vi "ROI grp-Add new POIs to the table.vi"(8 "error in (no error)":errorcluster, 11 "New POI indexes":i32[](array[numeric])) -> (0 "error out":errorcluster, 3 "reference out":refnum<vi>)   [LabVIEW 2020]
uses:
  Globals/gl_ROI grp window globals.vi
  <userlib>/_OpenG.lib/array/array.llb/Search 1D Array (String)__ogtk.vi
  <userlib>/_OpenG.lib/array/array.llb/Delete Elements from 1D Array (String)__ogtk.vi
panel:
  out "New number of rows":i32
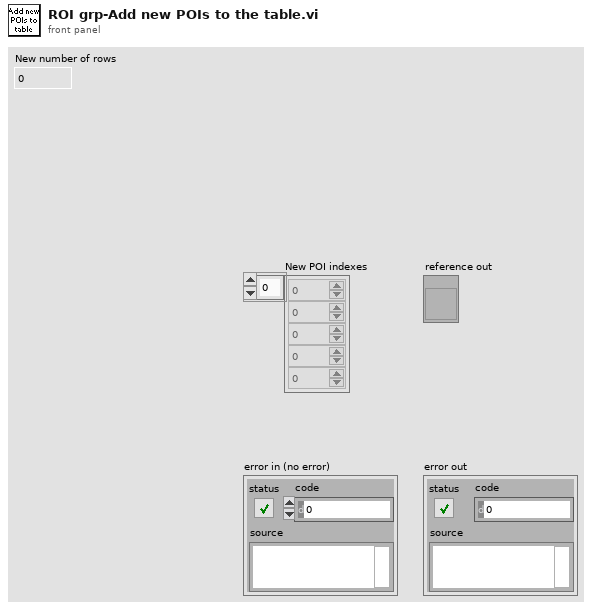
[diagram p1: front panel]
types:
  T1 = typedef "ROI grp-window ctrl refs.ctl" = cluster{"This VI":refnum<vi>, "Pane":refnum<vi>, "Table":refnum<vi>}
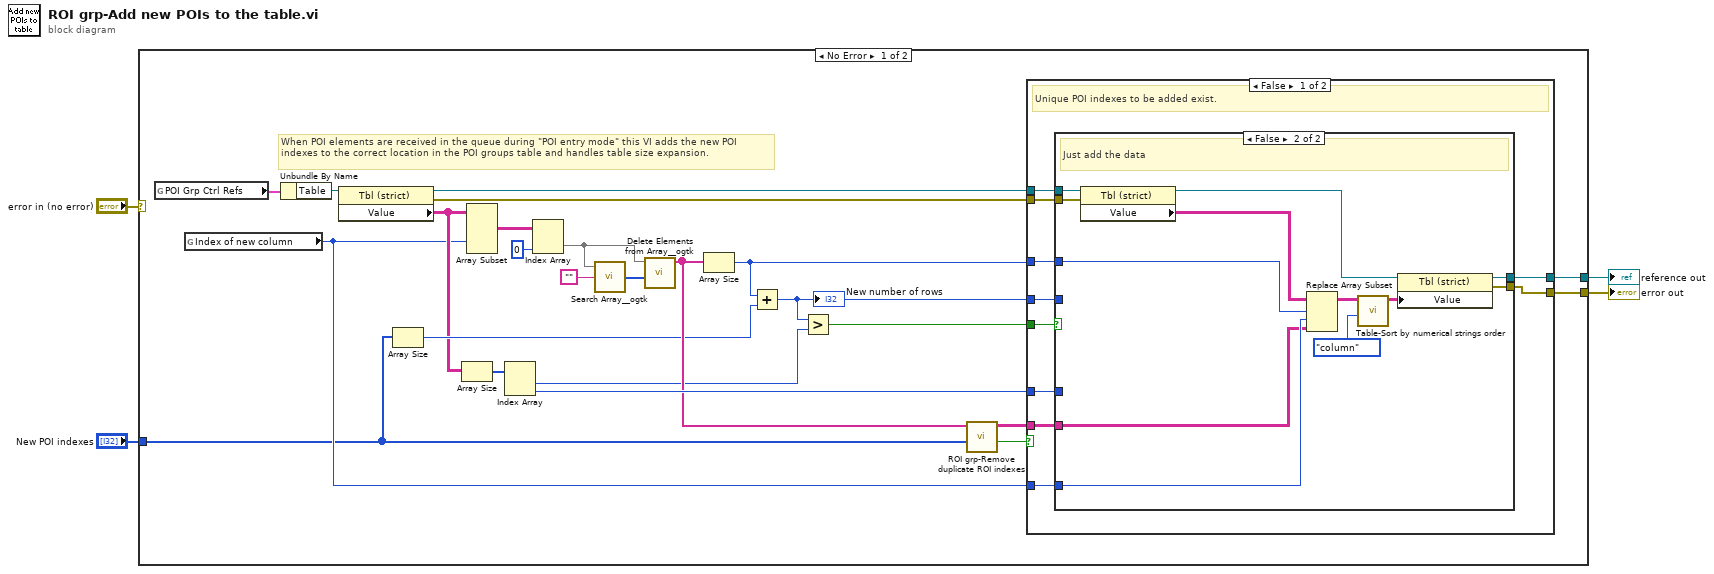
[diagram p0: block diagram]
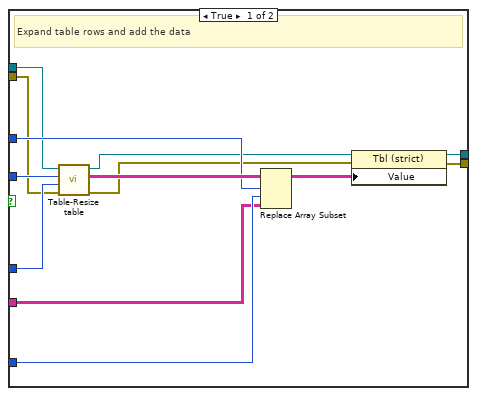
[diagram p2: hidden frame]
diagram:
  n1 = case shown="No Error" "error in (no error)" {
    selector: "error in (no error)" -> [_ w66]
    tunnel: [w11 _] -> w4
    tunnel: [w9 w66] -> w3
    tunnel: "New POI indexes" -> [w7 _]
    frame No Error {
      # "When POI elements are received in the queue during \"POI entry mode\" this VI adds the new POI indexes to the correct location in the POI groups table and handles table size expansion."
      n2 = global read "gl_ROI grp window globals.vi" "POI Grp Ctrl Refs"() -> (w5:T1)
      n3 = global read "gl_ROI grp window globals.vi" "Index of new column"() -> (w10:i32)
      n4 = Unbundle By Name(w5) -> ("Table"=w13:refnum<vi>)
      n5 = property class="Tbl (strict)"(reference=w13) -> (reference out=w12:refnum<vi>, error out=w14:errorcluster, "Value"=w17:string[][])  [unwired: 1 in]
      n6 = Array Size(array=w7) -> (size(s)=w21:i32)
      n7 = Array Size(array=w17) -> (size(s)=w26:i32[])
      n8 = Array Subset(array=w17, index (col)=w10) -> (w25:string[][])  [unwired: 3 in]
      n9 = Index Array(array=w26) -> (element #1=w20:i32, element #2=w28:i32)  [unwired: 2 in]
      n10 = Index Array(array=w25, index (col)=0 ("disabled index (col)")) -> (element=w16:string[])  [unwired: 1 in]
      n11 = call-poly <userlib>:"Search Array__ogtk.vi"("Array"=w16, "Element Data"="") -> ("Indices of Elements"=w23:i32[])  [unwired: 7 in]
      n12 = call-poly <userlib>:"Delete Elements from Array__ogtk.vi"("indices"=w23, "array"=w16) -> ("array w/ subset deleted"=w27:string[])  [unwired: 8 in, 1 out]
      n13 = Array Size(array=w27) -> (size(s)=w15:i32)
      n14 = Add(x=w15, y=w21) -> (x+y=w18:i32)
      "New number of rows" <- w18
      n15 = Greater?(x=w18, y=w20) -> (0:w19:bool)
      n16 = call "ROI grp-Remove duplicate ROI indexes.vi"("New POI indexes"=w7, "Current values in group to be edited"=w27) -> ("No unique new indexes to be added"=w6:bool, "New values that do not aldeady exist in the group"=w8:string[][])  [unwired: 8 in]
      n17 = case shown="False" w6 {
        tunnel: w19 -> [w38 _]
        tunnel: w18 -> [w37 _]
        tunnel: w28 -> [w36 _]
        tunnel: w15 -> [w35 _]
        tunnel: w14 -> [w34 w64]
        tunnel: w12 -> [w33 w65]
        tunnel: [w32 w65] -> w11
        tunnel: w10 -> [w31 _]
        tunnel: [w29 w64] -> w9
        tunnel: w8 -> [w30 _]
        frame False {
          # "Unique POI indexes to be added exist."
          n18 = case shown="False" w38 {
            tunnel: w37 -> [w51 _]
            tunnel: w36 -> [w50 _]
            tunnel: w33 -> [w45 w61]
            tunnel: w35 -> [w48 w63]
            tunnel: w34 -> [w46 w58]
            tunnel: [w43 w62] -> w32
            tunnel: w31 -> [w42 w57]
            tunnel: [w41 w56] -> w29
            tunnel: w30 -> [w39 w55]
            frame True {
              # "Expand table rows and add the data"
              n19 = call <userlib>:"Table-Resize table.vi"("error in (no error)"=w46, "Number of columns"=w50, "Number of rows"=w51, "Table ref in"=w45) -> ("error out"=w40:errorcluster, "Resized table"=w49:string[][], "Table ref out"=w44:refnum<vi>)  [unwired: 5 in]
              n20 = Replace Array Subset(array=w49, new element=w39, index (row)=w48, index (col)=w42) -> (w47:string[][])
              n21 = property class="Tbl (strict)"(reference=w44, error in=w40, "Value"=w47) -> (reference out=w43:refnum<vi>, error out=w41:errorcluster)
            }
            frame False {
              # "Just add the data"
              n22 = property class="Tbl (strict)"(reference=w61, error in=w58) -> (reference out=w60:refnum<vi>, "Value"=w59:string[][])  [unwired: 1 out]
              n23 = Replace Array Subset(array=w59, new element=w55, index (row)=w63, index (col)=w57) -> (w53:string[][])
              n24 = call <userlib>:"Table-Sort by numerical strings order.vi"("Sort By in"=enum16{"row", "column"}."column", "Numerical strings table in"=w53) -> ("Sorted numerical strings table"=w52:string[][])  [unwired: 8 in, 1 out]
              n25 = property class="Tbl (strict)"(reference=w60, "Value"=w52) -> (reference out=w62:refnum<vi>, error out=w56:errorcluster)  [unwired: 1 in]
            }
          }
        }
        frame True {
          # "No unique new indexes to be added"
        }
      }
    }
    frame Error {
    }
  }
  "reference out" <- w4
  "error out" <- w3
